vi "MISC Multiple Find and Replace.vi"(9 "Replace Text Array":string[](array[string]), 10 "Search Text Array":string[](array[string]), 11 "Input String":string) -> (1 "Match":bool, 2 "Matches":bool[](array[boolean]), 3 "Output String":string)   [LabVIEW 2017]
doc: "This routine performs a find and replace on each element pair in the search and replace arrays."
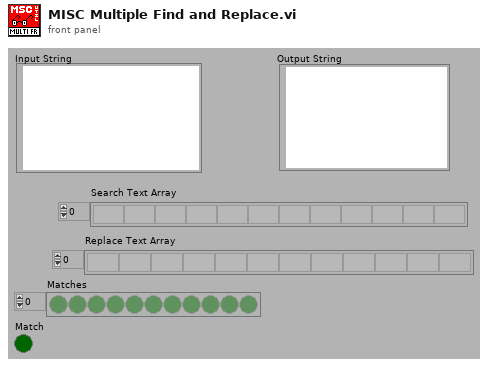
[diagram p1: front panel]
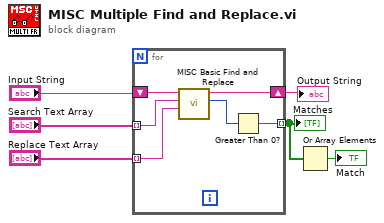
[diagram p0: block diagram]
diagram:
  n1 = for {
    tunnel: "Search Text Array" -> [w10] mode=indexing
    tunnel: "Replace Text Array" -> [w9] mode=indexing
    shift-right: [w11] -> w3
    shift-left: "Input String" -> [w12]
    tunnel: [w8] -> w2 mode=indexing
    n2 = call "MISC Basic Find and Replace.vi"("Replace Text"=w9, "Search Text"=w10, "Input String"=w12) -> ("Matches"=w7:i32, "Output String"=w11:string)  [unwired: 2 in, 5 out]
    n3 = Greater Than 0?(x=w7) -> (x > 0?=w8:bool)
  }
  "Output String" <- w3
  "Matches" <- w2
  n4 = Or Array Elements(Boolean array=w2) -> (logical OR=→"Match":bool)
